vi "Main - Computer.vi"() -> ()   [LabVIEW 2019]
uses:
  <vilib>/Utility/error.llb/DialogType.ctl
  <vilib>/DAQmx/read.llb/DAQmx Read (Analog 2D DBL NChan NSamp).vi
  <vilib>/Analysis/baseanly.llb/A x Vector.vi
  <vilib>/Analysis/1siggen.llb/Ramp Pattern by Samples.vi
  <vilib>/DAQmx/create/channels.llb/DAQmx Create Channel (AI-Voltage-Basic).vi
  <vilib>/DAQmx/configure/timing.llb/DAQmx Timing (Sample Clock).vi
  <vilib>/DAQmx/miscellaneous.llb/DAQmx Fill In Error Info.vi
  <vilib>/Utility/file.llb/Write To Spreadsheet File (DBL).vi
  <vilib>/Analysis/NI_AALBase.lvlib
panel:
  out "Logging":bool
  in  "Manual Logging":bool
  out "Force Units 2":string
  out "Torque Units 2":string
  in  "Transform":T1={"Dx"=0.0, "Dy"=0.0, "Dz"=0.0, "Rx"=90.0, "Ry"=-135.0, "Rz"=-90.0}
  in  "Calibration File":path=path "C:/Users/Hadrien Sprumont/Downloads/Installers/FT41361/FT41361.cal"
  in  "stop":bool
  out "Measurement":dbl[][](graph)
  in  "Log File":path=path "C:/Users/Hadrien Sprumont/Desktop/Soft Fish Experiments/Controller data/FT_sensor_data/test.csv"
  # "convertToFt"
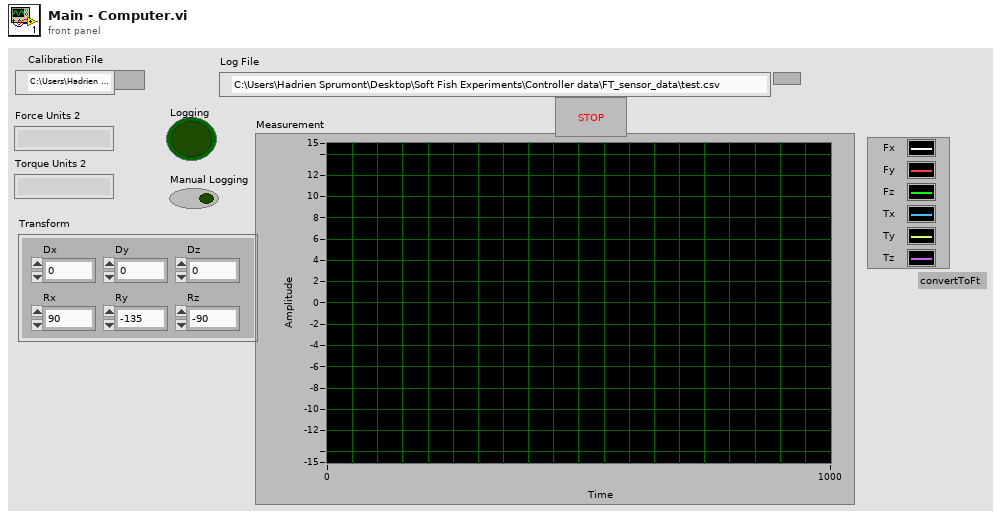
[diagram p1: front panel]
types:
  T1 = cluster{"Dx":dbl, "Dy":dbl, "Dz":dbl, "Rx":dbl, "Ry":dbl, "Rz":dbl}
  T2 = typedef "DialogType.ctl" = u16
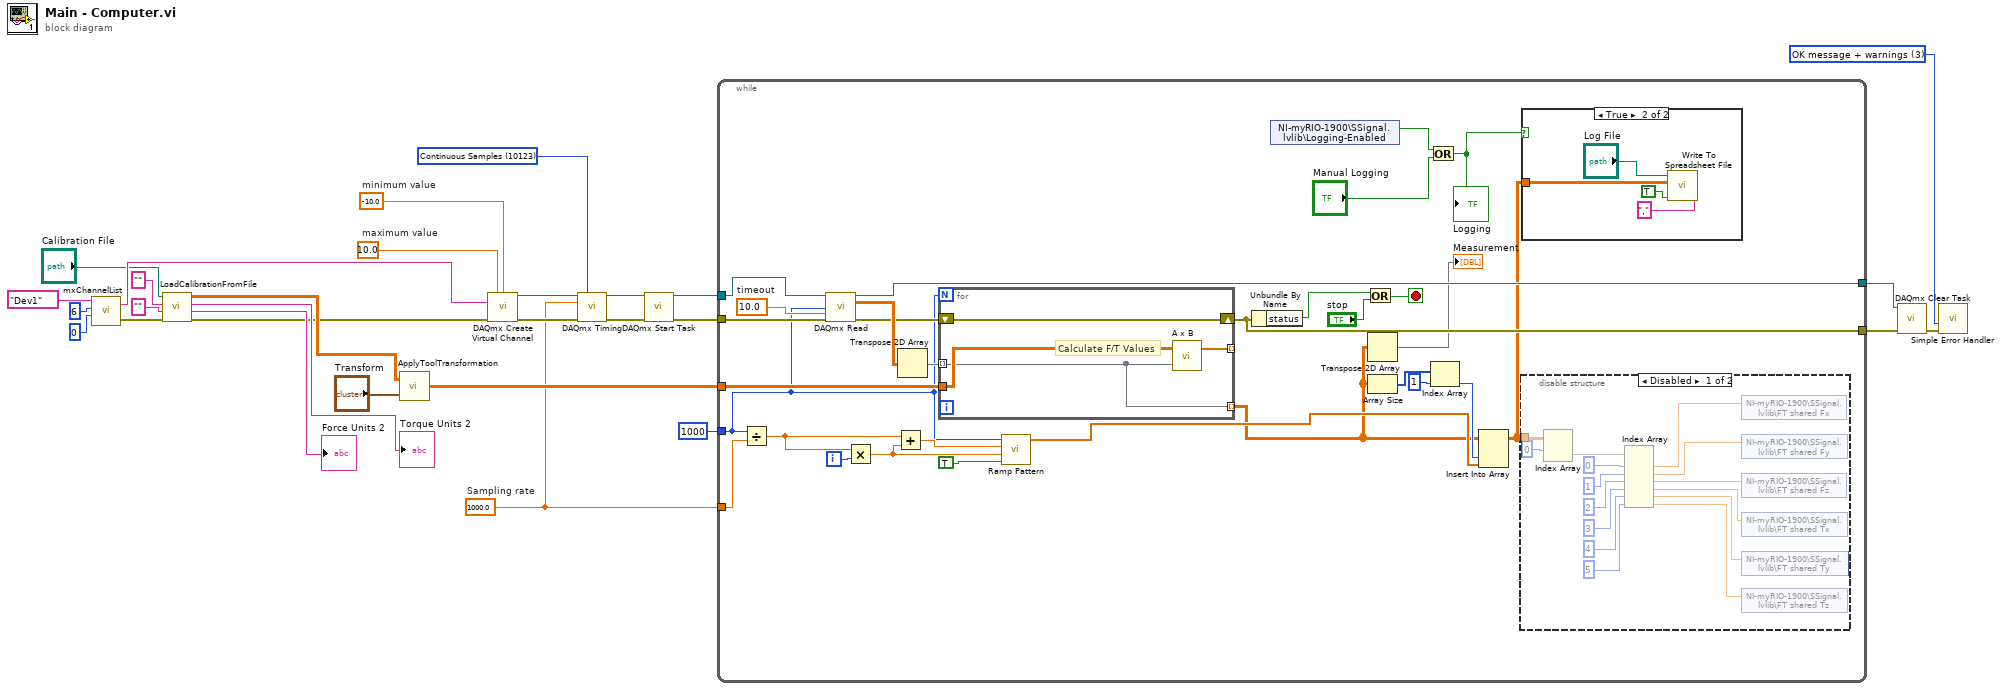
[diagram p0: block diagram]
diagram:
  w2 = 1000.0  # Sampling rate
  w3 = -10.0  # minimum value
  w4 = 10.0  # maximum value
  w22 = T2 3 items=["no dialog", "OK message", "continue or stop message", "OK message + warnings", "continue/stop + warnings"] ("type of dialog (OK msg:1)")
  w24 = 10123 items=["Finite Samples"=10178, "Continuous Samples"=10123] ("sample mode")
  n1 = call "mxChannelList.vi"("First Channel"=i16 0, "Number of Channels"=6, "DAQmx Device Name"=tag "Dev1") -> ("error out"=w9:errorcluster, "Channel List"=w19:string)  [unwired: 1 in]
  n2 = call "LoadCalibrationFromFile.vi"("Error In"=w9, "User Torque Units"="", "User Force Units"="", "Cal File Path"="Calibration File") -> ("Error Out"=w8:errorcluster, "Calibration Force Units"=→"Force Units 2":string, "Calibration Torque Units"=→"Torque Units 2":string, "Calibration Matrix"=w13:dbl[][])
  n3 = call "ApplyToolTransformation.vi"("Transform"="Transform", "Calibration Matrix"=w13) -> ("Transformed Calibration Matrix"=w12:dbl[][])
  n4 = call-poly <vilib>:"DAQmx Create Virtual Channel.vi"("maximum value"=w4, "minimum value"=w3, "physical channels"=w19, "error in"=w8) -> ("task out"=w27:refnum<k21>, "error out"=w29:errorcluster)  [unwired: 10 in]
  n5 = call-poly <vilib>:"DAQmx Timing.vi"("task/channels in"=w27, "sample mode"=w24, "rate"=w2, "error in"=w29) -> ("task out"=w23:refnum<k21>, "error out"=w18:errorcluster)  [unwired: 10 in]
  n6 = call <vilib>:"DAQmx Start Task.vi"("task/channels in"=w23, "error in"=w18) -> ("task out"=w26:refnum<k21>, "error out"=w17:errorcluster)  [unwired: 12 in]
  n7 = while {
    tunnel: w26 -> [w58]
    tunnel: [w57] -> w25
    tunnel: w17 -> [w38]
    tunnel: [w37] -> w16
    tunnel: w12 -> [w52]
    tunnel: w2 -> [w48]
    tunnel: 1000 ("samples") -> [w35]
    i -> [w47]
    stop <- w53 stop-if-true
    w56 = 10.0  # timeout
    n8 = Divide(x=w35, y=w48) -> (x/y=w46:dbl)
    n9 = call-poly <vilib>:"DAQmx Read.vi"("task/channels in"=w58, "number of samples per channel"=w35, "timeout"=w56, "error in"=w38) -> ("task out"=w57:refnum<k21>, "data"=w50:dbl[][], "error out"=w39:errorcluster)  [unwired: 9 in]
    n10 = Multiply(x=w46, y=w47) -> (x*y=w44:dbl)
    n11 = Add(x=w46, y=w44) -> (x+y=w45:dbl)
    n12 = Transpose 2D Array(2D array=w50) -> (transposed array=w51:dbl[][])
    n13 = for {
      N: w35 -> [_]
      tunnel: [w81] -> _ mode=indexing
      shift-right: [w80] -> w37
      shift-left: w39 -> [w80]
      tunnel: w51 -> [w78] mode=indexing
      tunnel: w52 -> [w79]
      tunnel: [w78] -> w31 mode=indexing
      # "Calculate F/T Values"
      n14 = call-poly <vilib>:"A x B.vi"("Vector"=w78, "A"=w79) -> ("A x Vector"=w81:dbl[])  [unwired: 1 out]
    }
    n15 = call-poly <vilib>:"Ramp Pattern.vi"("exclude end?"=TRUE, "start"=w44, "end"=w45, "samples"=w35) -> ("Ramp Pattern"=w43:dbl[])  [unwired: 6 in, 1 out]
    n16 = Unbundle By Name(w37) -> ("status"=w54:bool)
    n17 = shared-variable "NI-myRIO-1900\\SSignal.lvlib\\Logging-Enabled"() -> (w32:bool)  [unwired: 1 in, 1 out]
    n18 = Or(x=w54, y="stop") -> (x .or. y?=w53:bool)
    n19 = Transpose 2D Array(2D array=w31) -> (transposed array=→"Measurement":dbl[][])
    n20 = Array Size(array=w31) -> (size(s)=w41:i32[])
    n21 = Or(x=w32, y="Manual Logging") -> (x .or. y?=w34:bool)
    "Logging" <- w34
    n22 = Index Array(array=w41, index=1) -> (element=w40:i32)
    n23 = Insert Into Array(array=w31, index (col)=w40, new element=w43) -> (w36:dbl[][])  [unwired: 1 in]
    n24 = disable-structure shown="Disabled" {
      disable-tunnel: w36 -> [w73 _]
      frame Disabled {
        n25 = Index Array(array=w73, index (row)=0) -> (element=w71:dbl[])  [unwired: 1 in]
        n26 = Index Array(array=w71, index #1=0 ("index"), index #2=1 ("index"), index #3=2 ("index"), index #4=3 ("index"), index #5=4 ("index"), index #6=5 ("index")) -> (element #1=w63:dbl, element #2=w62:dbl, element #3=w61:dbl, element #4=w60:dbl, element #5=w59:dbl, element #6=w64:dbl)
        n27 = shared-variable "NI-myRIO-1900\\SSignal.lvlib\\FT shared Fx"(w63) -> ()  [unwired: 1 in, 1 out]
        n28 = shared-variable "NI-myRIO-1900\\SSignal.lvlib\\FT shared Fy"(w62) -> ()  [unwired: 1 in, 1 out]
        n29 = shared-variable "NI-myRIO-1900\\SSignal.lvlib\\FT shared Fz"(w61) -> ()  [unwired: 1 in, 1 out]
        n30 = shared-variable "NI-myRIO-1900\\SSignal.lvlib\\FT shared Tx"(w60) -> ()  [unwired: 1 in, 1 out]
        n31 = shared-variable "NI-myRIO-1900\\SSignal.lvlib\\FT shared Ty"(w59) -> ()  [unwired: 1 in, 1 out]
        n32 = shared-variable "NI-myRIO-1900\\SSignal.lvlib\\FT shared Tz"(w64) -> ()  [unwired: 1 in, 1 out]
      }
      frame Enabled {
      }
    }
    n33 = case shown="True" w34 {
      tunnel: w36 -> [_ w77]
      frame False {
      }
      frame True {
        n34 = call-poly <vilib>:"Write To Spreadsheet File.vi"("delimiter (\\t)"=",", "append to file? (new file:F)"=TRUE, "2D data"=w77, "file path (dialog if empty)"="Log File") -> ()  [unwired: 4 in, 1 out]
      }
    }
  }
  n35 = call <vilib>:"DAQmx Clear Task.vi"("task in"=w25, "error in"=w16) -> ("error out"=w28:errorcluster)  [unwired: 13 in]
  n36 = call <vilib>:"Simple Error Handler.vi"("type of dialog (OK msg:1)"=w22, "error in (no error)"=w28) -> ()  [unwired: 3 in, 5 out]
